vi "meTEC_Find TECs.vi"(8 "error in (no error)":errorcluster, 11 "VISA Resources List (COM Ports)":string[](array[string])) -> (0 "error out":errorcluster, 3 "VISA Resources List (meTEC(s))":string[](array[string]))   [LabVIEW 2019]
uses:
  TypeDefs/meTEC_Configuration.ctl
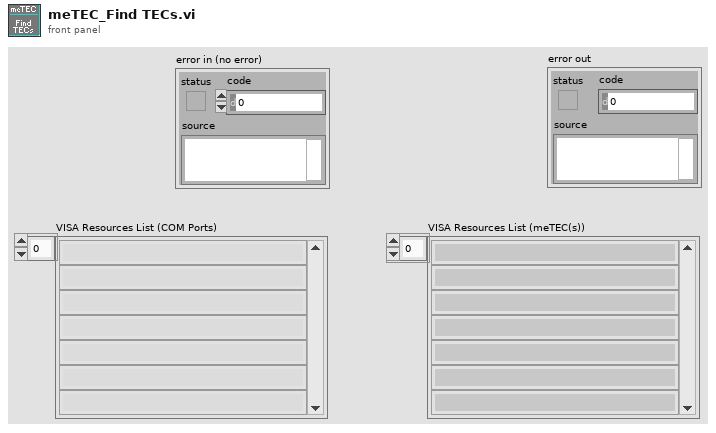
[diagram p1: front panel]
types:
  T1 = typedef "meTEC_Configuration.ctl" = cluster{"VISA resource name":refnum<visa-resource-name>, "Device Address":u16}
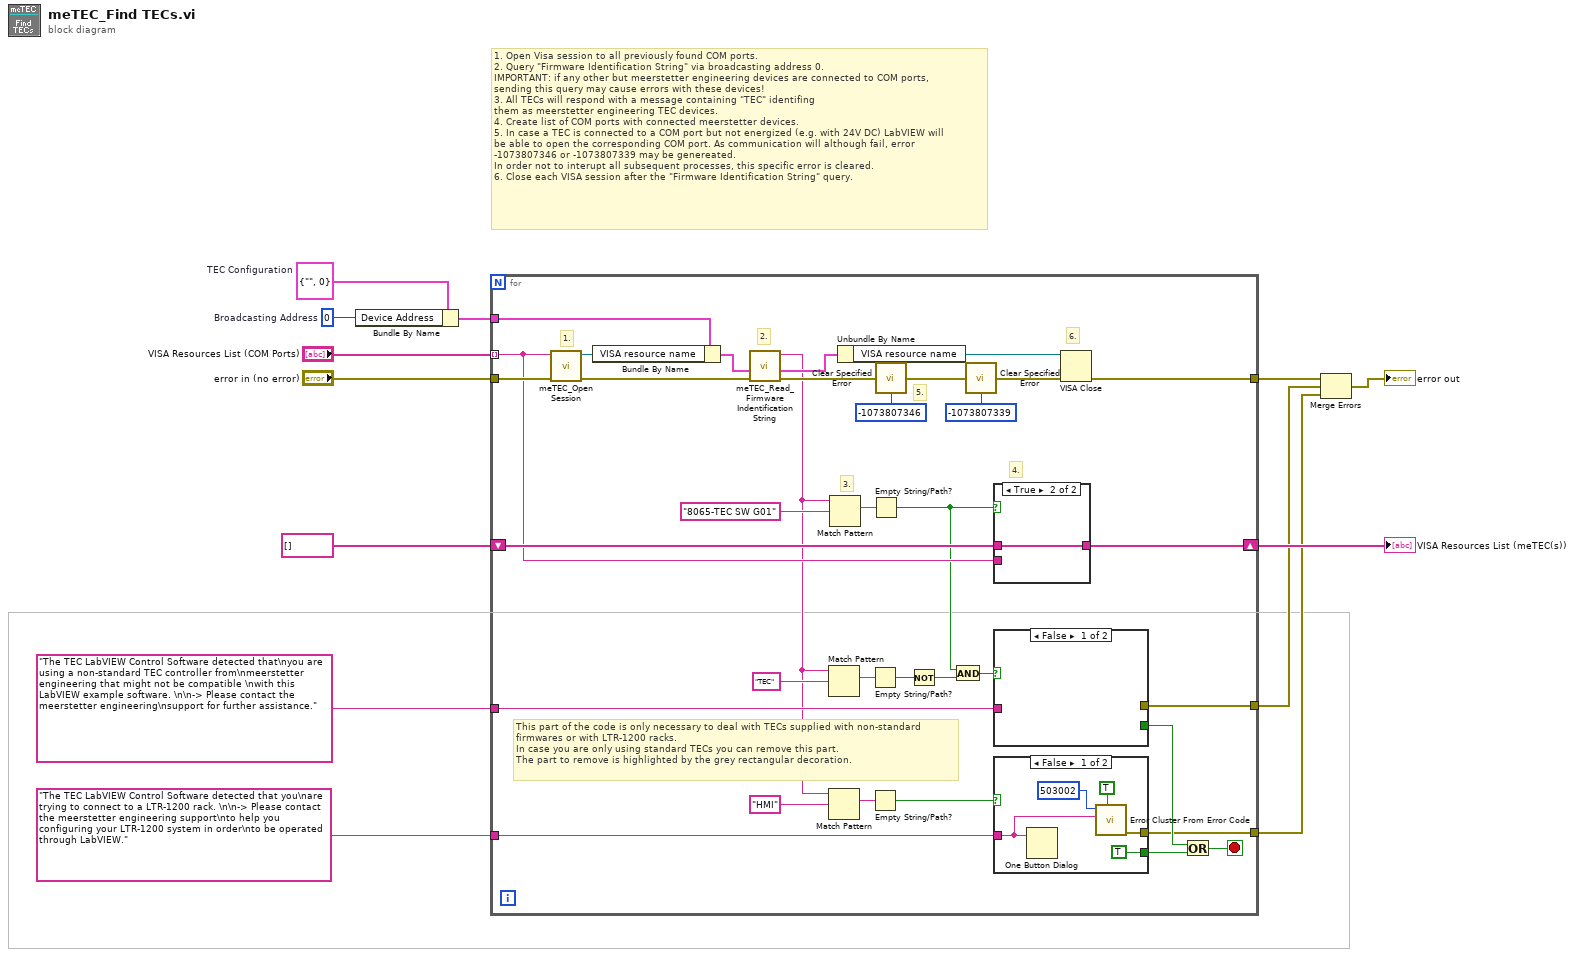
[diagram p0: block diagram]
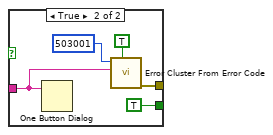
[diagram p3: hidden frame]
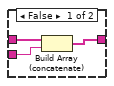
[diagram p4: hidden frame]
diagram:
  w8 = u16 0  # Broadcasting Address
  w9 = T1 {"VISA resource name"="", "Device Address"=0}  # TEC Configuration
  # "1. Open Visa session to all previously found COM ports.\n2. Query \"Firmware Identification String\" via broadcasting address 0.\nIMPORTANT: if any other but meerstetter engineering devices are connected to COM ports, \nsending this query may cause errors with these devices!\n3. All TECs will respond with a message containing \"TEC\" identifing\nthem as meerstetter engineering TEC devices.\n4. Create list of COM ports with connected meerstetter devices.\n5. In case a TEC is connected to a COM port but not energized (e.g. with 24V DC) LabVIEW will\nbe able to open the corresponding COM port. As communication will although fail, error \n-1073807346 or -1073807339 may be genereated.\nIn order not to interupt all subsequent processes, this specific error is cleared. \n6. Close each VISA session after the \"Firmware Identification String\" query."
  n1 = Bundle By Name(cluster=w9, "Device Address"=w8) -> (w7:T1)
  n2 = for {
    tunnel: [w48] -> w5
    tunnel: "error in (no error)" -> [w42]
    tunnel: "VISA Resources List (COM Ports)" -> [w40] mode=indexing
    shift-right: [w45] -> w10
    shift-left: string[] [] -> [w44]
    tunnel: w7 -> [w38]
    tunnel: "The TEC LabVIEW Control Software detected that\nyou are using a non-standard TEC controller from\nmeerstetter engineering that might not be compatible \nwith this LabVIEW example software. \n\n-> Please contact the meerstetter engineering\nsupport for further assistance." ("regular expression") -> [w26]
    tunnel: [w25] -> w3
    tunnel: "The TEC LabVIEW Control Software detected that you\nare trying to connect to a LTR-1200 rack. \n\n-> Please contact the meerstetter engineering support\nto help you configuring your LTR-1200 system in order\nto be operated through LabVIEW." ("regular expression") -> [w22]
    tunnel: [w16] -> w1
    stop <- w24 stop-if-true
    # "This part of the code is only necessary to deal with TECs supplied with non-standard\nfirmwares or with LTR-1200 racks.\nIn case you are only using standard TECs you can remove this part.\nThe part to remove is highlighted by the grey rectangular decoration."
    # "6."
    # "5."
    # "4."
    # "3."
    # "2."
    # "1."
    n3 = call "meTEC_Open Session.vi"("error in (no error)"=w42, "COM Port"=w40) -> ("error out"=w41:errorcluster, "VISA resource name_OUT"=w37:refnum<visa-resource-name>)  [unwired: 8 in]
    n4 = Bundle By Name(cluster=w38, "VISA resource name"=w37) -> (w36:T1)
    n5 = call "meTEC_Read_Firmware Indentification String.vi"("error in (no error)"=w41, "TEC Configuration_IN"=w36) -> ("error out"=w43:errorcluster, "TEC Configuration_OUT"=w35:T1, "Firmware Identification String"=w19:string)  [unwired: 7 in]
    n6 = Match Pattern(string=w19, regular expression="TEC") -> (match substring=w30:string)  [unwired: 1 in, 3 out]
    n7 = Match Pattern(string=w19, regular expression="HMI") -> (match substring=w20:string)  [unwired: 1 in, 3 out]
    n8 = Match Pattern(string=w19, regular expression="8065-TEC SW G01") -> (match substring=w46:string)  [unwired: 1 in, 3 out]
    n9 = Unbundle By Name(w35) -> ("VISA resource name"=w39:refnum<visa-resource-name>)
    n10 = Empty String/Path?(string/path=w30) -> (empty?=w27:bool)
    n11 = Empty String/Path?(string/path=w20) -> (empty?=w17:bool)
    n12 = Empty String/Path?(string/path=w46) -> (empty?=w15:bool)
    n13 = call "Clear Specified Error.vi"("error in (no error)"=w43, "Code to Clear (0)"=-1073807346) -> ("error out"=w32:errorcluster)
    n14 = Not(x=w27) -> (.not. x?=w14:bool)
    n15 = And(x=w15, y=w14) -> (x .and. y?=w28:bool)
    n16 = call "Clear Specified Error.vi"("error in (no error)"=w32, "Code to Clear (0)"=-1073807339) -> ("error out"=w31:errorcluster)
    n17 = case shown="True" w15 {
      tunnel: w40 -> [w61 _]
      tunnel: [w60 w62] -> w45
      tunnel: w44 -> [w59 w62]
      frame False {
        n18 = Build Array (concatenate)(w59, w61) -> (w60:string[])
      }
      frame True {
      }
    }
    n19 = case shown="False" w28 {
      tunnel: w26 -> [_ w58]
      tunnel: [_ w55] -> w25
      tunnel: [_ TRUE ("show call chain? (False)")] -> w23
      frame False {
      }
      frame True {
        n20 = One Button Dialog(message=w58) -> ()  [unwired: 1 in, 1 out]
        n21 = call <vilib>:"Error Cluster From Error Code.vi"("show call chain? (False)"=TRUE, "error message (\"\")"=w58, "error code (0)"=503001) -> ("error out"=w55:errorcluster)  [unwired: 6 in]
      }
    }
    n22 = case shown="False" w17 {
      tunnel: w22 -> [w53 _]
      tunnel: [w50 _] -> w16
      tunnel: [TRUE ("show call chain? (False)") _] -> w18
      frame False {
        n23 = One Button Dialog(message=w53) -> ()  [unwired: 1 in, 1 out]
        n24 = call <vilib>:"Error Cluster From Error Code.vi"("show call chain? (False)"=TRUE, "error message (\"\")"=w53, "error code (0)"=503002) -> ("error out"=w50:errorcluster)  [unwired: 6 in]
      }
      frame True {
      }
    }
    n25 = VISA Close(VISA resource name=w39, error in (no error)=w31) -> (error out=w48:errorcluster)
    n26 = Or(x=w23, y=w18) -> (x .or. y?=w24:bool)
  }
  "VISA Resources List (meTEC(s))" <- w10
  n27 = Merge Errors(w5, w3, w1) -> (→"error out":errorcluster)
